vi "Settings Page.vi"() -> ()   [LabVIEW 2018, in "Protocols.lvlib" / "UDP.lvclass"]
uses:
  UDP.lvclass
panel:
  in  "Protocol Settings":enum32{"UDP"}(tab)
  in  "UDP Browse":bool
  in  "Target Port":u16
  in  "Target IP Address":string="localhost"
  in  "Local Port":u16
  in  "Local IP Address":string="localhost"
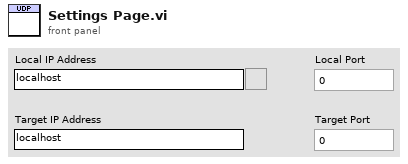
[diagram p1: front panel]
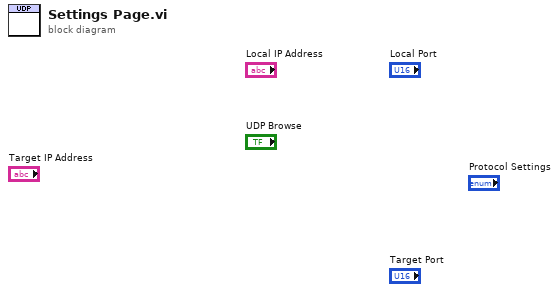
[diagram p0: block diagram]
diagram:
